vi "Fetch Class Methods Info.vi"(5 "Parser Settings":T9, 8 "Error in":errorcluster caption="Error in (no error)", 11 "LVClassLibrary":refnum<vi>) -> (0 "Error out":errorcluster, 2 "Methods":T1[](array[typedef]))   [LabVIEW 2023, in "VIDoc Parsing.lvlib"]
uses:
  VIDoc Parsing.lvlib
  Settings/Parser Settings/Parser Settings Cluster.ctl
  Settings/Parser Settings/Draw Controls Cluster.ctl
  Settings/Parser Settings/Draw Option Enum.ctl
  TypeDefs/Method Spec Cluster.ctl
  TypeDefs/VI Type Extended Enum.ctl
  <vilib>/picture/picture.llb/imagedata.ctl
  TypeDefs/Class Dispatch Type Enum.ctl
  TypeDefs/Controls Info Cluster.ctl
  <vilib>/Utility/miscctls.llb/LVKeyTypeDef.ctl
  <vilib>/Utility/miscctls.llb/LVPointTypeDef.ctl
  Structure Reporter/Tree Cluster.ctl
  Structure Reporter/Structure Reporter.lvlib
  Settings/Parser Settings/Parser Settings.lvclass
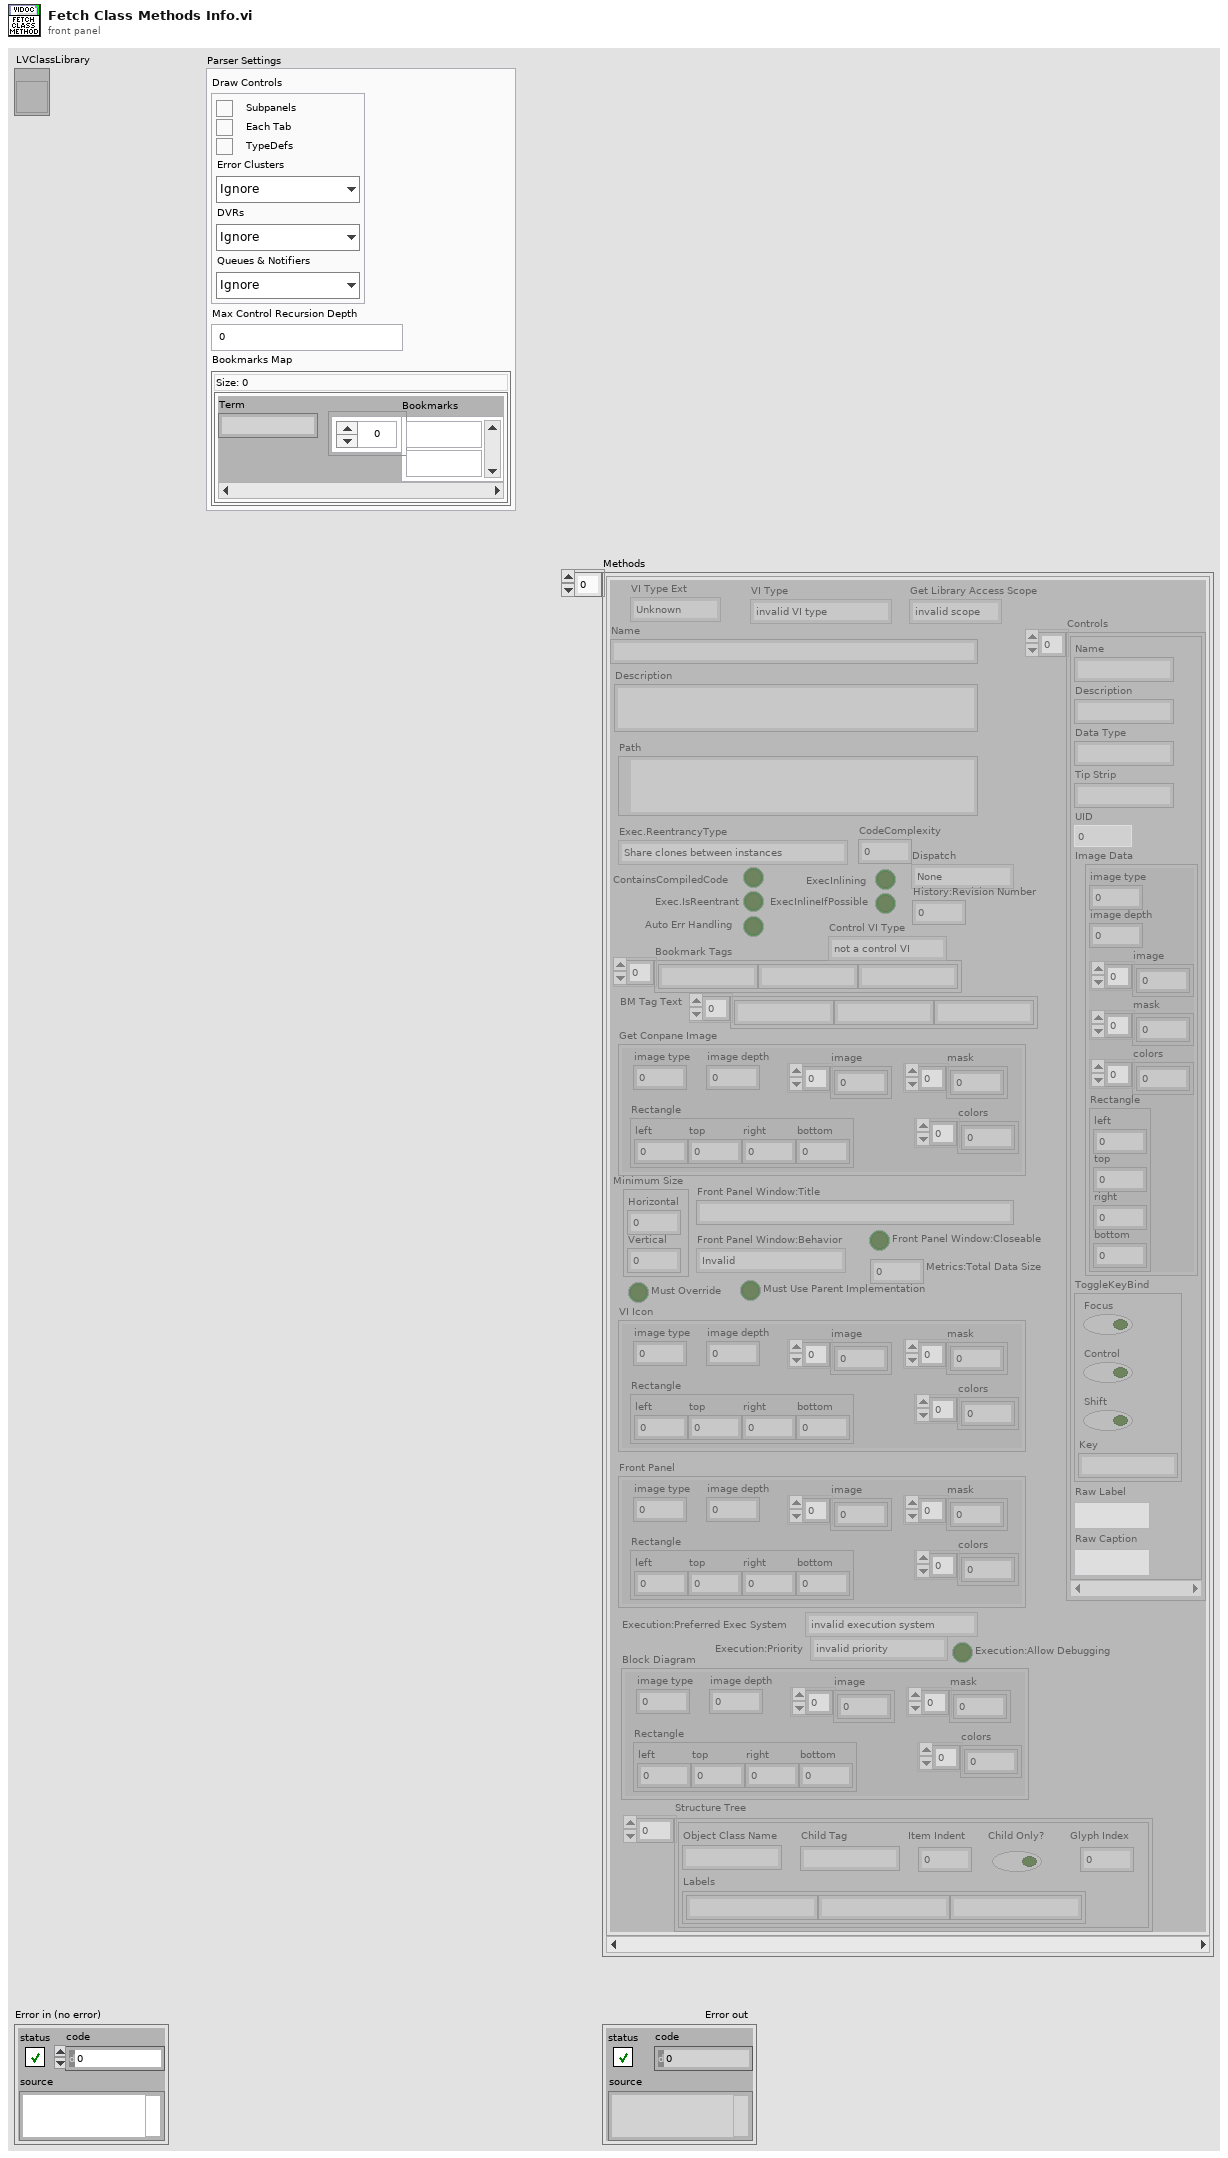
[diagram p1: front panel]
types:
  T1 = typedef "VIDoc Parsing.lvlib/Method Spec Cluster.ctl" = cluster{"VI Type Ext":T2, "Name":string, "Path":path, "Get Conpane Image":T3, "Description":string, "Get Library Access Scope":enum32{"invalid scope", "public", "private", "protected", "community"}, "Dispatch":T4, "ContainsCompiledCode":bool, "Exec.IsReentrant":bool, "Exec.ReentrancyType":enum16{"Share clones between instances", "Preallocate clone for each instance"}, "ExecInlining":bool, "ExecInlineIfPossible":bool, "Auto Err Handling":bool, "CodeComplexity":sgl, "Bookmark Tags":string[], "Control VI Type":enum32{"not a control VI", "control", "typedef", "strict typedef"}, "Controls":T5[], "VI Type":enum32{"invalid VI type", "Standard VI", "Control VI", "Global VI", "Polymorphic VI", "Configuration VI", "SubSystem", "Facade VI", "Method VI", "Statechart Diagram VI"}, "Minimum Size":T7, "Front Panel Window:Title":string, "Front Panel Window:Behavior":enum32{"Invalid", "Default", "Floating", "Floating/Auto-Hide", "Modal"}, "Front Panel Window:Closeable":bool, "Must Override":bool, "Must Use Parent Implementation":bool, "VI Icon":T3, "Front Panel":T3, "History:Revision Number":u32, "Metrics:Total Data Size":u32, "Execution:Allow Debugging":bool, "Execution:Preferred Exec System":enum32{"invalid execution system", "user interface", "standard", "instrument i/o", "data acquisition", "other 1", "other 2", "same as caller"}, "Execution:Priority":enum32{"invalid priority", "background priority", "normal priority", "above normal priority", "high priority", "time critical priority", "subroutine"}, "BM Tag Text":string[], "Block Diagram":T3, "Structure Tree":T8[]}
  T2 = typedef "VIDoc Parsing.lvlib/VI Type Extended Enum.ctl" = enum16{"Unknown", "Class Method", "Class Accessor Get", "Class Accessor Set", "Class Control", "Library Method", "Library Control", "VI", "Control"}
  T3 = typedef "imagedata.ctl" = cluster{"image type":i32, "image depth":i32, "image":u8[], "mask":u8[], "colors":u32[], "Rectangle":cluster{"left":i16, "top":i16, "right":i16, "bottom":i16}}
  T4 = typedef "VIDoc Parsing.lvlib/Class Dispatch Type Enum.ctl" = enum16{"None", "Static", "Dynamic"}
  T5 = typedef "VIDoc Parsing.lvlib/Controls Info Cluster.ctl" = cluster{"Name":string, "Description":string, "Data Type":string, "Tip Strip":string, "UID":i32, "Image Data":T3, "ToggleKeyBind":T6, "Raw Label":string, "Raw Caption":string}
  T6 = typedef "LVKeyTypeDef.ctl" = cluster{"Focus":bool, "Control":bool, "Shift":bool, "Key":string}
  T7 = typedef "LVPointTypeDef.ctl" = cluster{"Horizontal":i16, "Vertical":i16}
  T8 = typedef "VIDoc Parsing.lvlib/Structure Reporter.lvlib/Tree Cluster.ctl" = cluster{"Object Class Name":string, "Labels":string[], "Child Tag":string, "Item Indent":i32, "Child Only?":bool, "Glyph Index":i32}
  T9 = typedef "VIDoc Parsing.lvlib/Parser Settings.lvclass/Parser Settings Cluster.ctl" = cluster{"Draw Controls":T10, "Max Control Recursion Depth":i32, "Bookmarks Map":map{string, string[]}}
  T10 = typedef "VIDoc Parsing.lvlib/Parser Settings.lvclass/Draw Controls Cluster.ctl" = cluster{"Subpanels":bool, "Tabs":bool, "TypeDefs":bool, "Error Clusters":T11, "DVRs":T11, "Queues & Notifiers":T11}
  T11 = typedef "VIDoc Parsing.lvlib/Parser Settings.lvclass/Draw Option Enum.ctl" = enum16{"Ignore", "Draw", "Draw + Contents"}
  T12 = enum32{"invalid VI type", "Standard VI", "Control VI", "Global VI", "Polymorphic VI", "Configuration VI", "SubSystem", "Facade VI", "Method VI", "Statechart Diagram VI"}
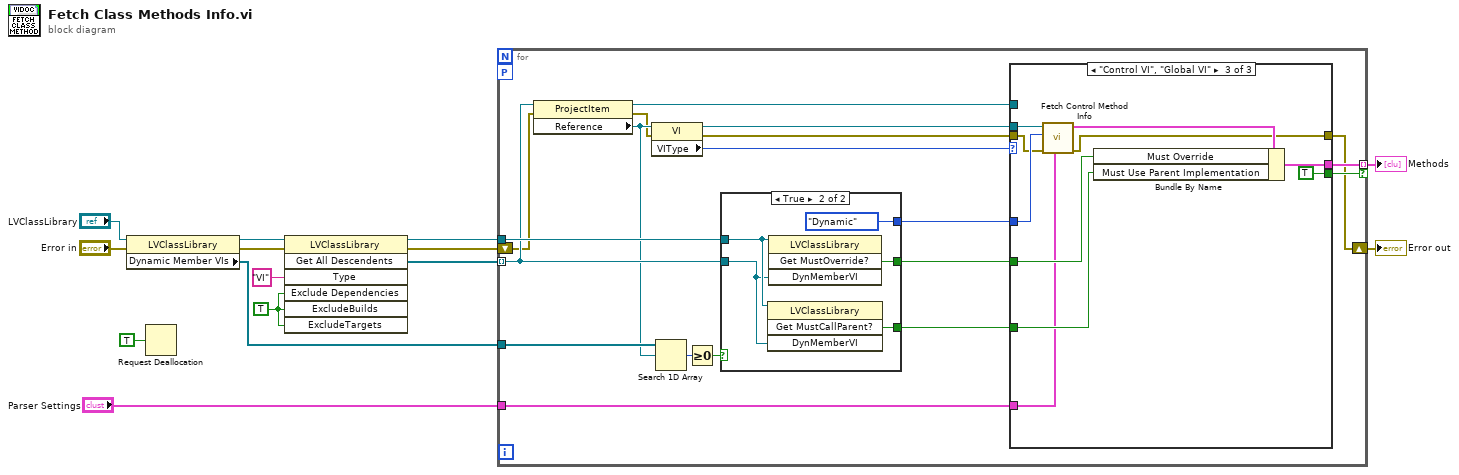
[diagram p0: block diagram]
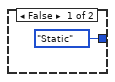
[diagram p2: hidden frame]
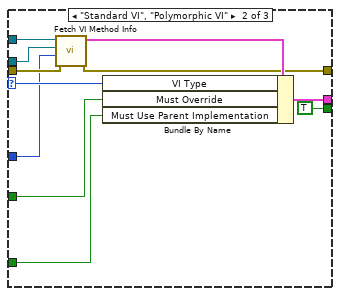
[diagram p4: hidden frame]
diagram:
  w8 = TRUE ("ExcludeDependencies")
  n1 = property class="LVClassLibrary"(reference="LVClassLibrary", error in="Error in") -> (reference out=w11:refnum<vi>, error out=w9:errorcluster, "Dynamic Member VIs"=w4:refnum<vi>[])
  n2 = Request Deallocation(TRUE ("flag")) -> ()
  n3 = invoke class="LVClassLibrary" method="Get All Descendents"(reference=w11, error in=w9, "Type"="VI", "Exclude Dependencies"=w8, "ExcludeBuilds"=w8, "ExcludeTargets"=w8) -> (reference out=w7:refnum<vi>, error out=w3:errorcluster, "All Descendents"=w6:refnum<vi>[])  [unwired: 1 in, 4 out]
  n4 = for {
    tunnel: w4 -> [w25]
    tunnel: [w31] -> w5 mode=indexing if=w30
    tunnel: w7 -> [w29]
    tunnel: w6 -> [w24] mode=indexing
    shift-right: [w16] -> w2
    shift-left: w3 -> [w19]
    tunnel: "Parser Settings" -> [w15]
    workers-P: _ -> [_]
    n5 = property class="ProjectItem"(reference=w24, error in=w19) -> (reference out=w28:refnum<vi>, error out=w18:errorcluster, "Reference"=w23:refnum<vi>)
    n6 = property class="VI"(reference=w23, error in=w18) -> (reference out=w32:refnum<vi>, error out=w17:errorcluster, "VIType"=w33:T12)
    n7 = Search 1D Array(1D array=w25, element=w23) -> (index of element=w22:i32)  [unwired: 1 in]
    n8 = Greater Or Equal To 0?(x=w22) -> (x >= 0?=w21:bool)
    n9 = case shown="True" w21 {
      tunnel: w29 -> [_ w39]
      tunnel: w24 -> [_ w38]
      tunnel: [_ w37] -> w26
      tunnel: [_ w36] -> w27
      tunnel: [Class_Dispatch_Type_Enum."Static" Class_Dispatch_Type_Enum."Dynamic"] -> w20
      frame False {
      }
      frame True {
        n10 = invoke class="LVClassLibrary" method="Get MustCallParent?"(reference=w39, "DynMemberVI"=w38) -> ("Get MustCallParent?"=w36:bool)  [unwired: 2 in, 3 out]
        n11 = invoke class="LVClassLibrary" method="Get MustOverride?"(reference=w39, "DynMemberVI"=w38) -> ("GetMustOverride"=w37:bool)  [unwired: 2 in, 3 out]
      }
    }
    n12 = case shown="\"Control VI\", \"Global VI\"" w33 {
      selector: w33 -> [_ w50 _]
      tunnel: w32 -> [_ w41 w56]
      tunnel: w20 -> [_ w42 w55]
      tunnel: w28 -> [_ w46 _]
      tunnel: [_ w49 w58] -> w31
      tunnel: [_ TRUE TRUE] -> w30
      tunnel: w26 -> [_ w48 w60]
      tunnel: w27 -> [_ w47 w59]
      tunnel: w17 -> [w40 w44 w54]
      tunnel: [w40 w43 w53] -> w16
      tunnel: w15 -> [_ _ w52]
      frame Default {
      }
      frame "Standard VI", "Polymorphic VI" {
        n13 = call "Fetch VI Method Info.vi"("Error in"=w44, "Dispatch (None)"=w42, "VI Reference"=w41, "VI ProjectItem in"=w46) -> ("Error out"=w43:errorcluster, "Method Spec Cluster"=w45:T1)  [unwired: 6 in]
        n14 = Bundle By Name(cluster=w45, "VI Type"=w50, "Must Override"=w48, "Must Use Parent Implementation"=w47) -> (w49:T1)
      }
      frame "Control VI", "Global VI" {
        n15 = call "Fetch Control Method Info.vi"("Parser Settings"=w52, "Error in"=w54, "Dispatch (None)"=w55, "VI in"=w56) -> ("Error out"=w53:errorcluster, "Method Spec Cluster"=w57:T1)  [unwired: 6 in]
        n16 = Bundle By Name(cluster=w57, "Must Override"=w60, "Must Use Parent Implementation"=w59) -> (w58:T1)
      }
    }
  }
  "Error out" <- w2
  "Methods" <- w5
